vi "dfd_Build Filter Name.vi"(1 "filter name in":string) -> (0 "filter name out":string)   [LabVIEW 2017, in "NI_DigFilterLicensed.lvlib"]
uses:
  <vilib>/addons/Digital Filter Design/NI_DigFilterLicensed.lvlib
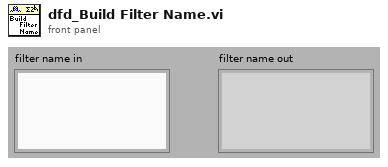
[diagram p1: front panel]
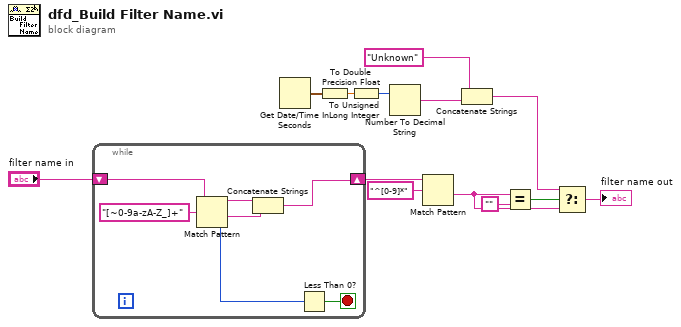
[diagram p0: block diagram]
diagram:
  n1 = while {
    shift-right: [w16] -> w3
    shift-left: "filter name in" -> [w20]
    stop <- w15 stop-if-true
    n2 = Match Pattern(string=w20, regular expression="[~0-9a-zA-Z_]+") -> (before substring=w18:string, after substring=w17:string, offset past match=w14:i32)  [unwired: 2 out]
    n3 = Concatenate Strings(w18, w17) -> (w16:string)
    n4 = Less Than 0?(x=w14) -> (x < 0?=w15:bool)
  }
  n5 = Get Date/Time In Seconds() -> (seconds since 1Jan1904=w10:timestamp)
  n6 = To Double Precision Float(number=w10) -> (double precision float=w9:dbl)
  n7 = To Unsigned Long Integer(number=w9) -> (unsigned 32bit integer=w8:u32)
  n8 = Number To Decimal String(number=w8) -> (decimal integer string=w7:string)  [unwired: 1 out]
  n9 = Match Pattern(string=w3, regular expression="^[0-9]*") -> (after substring=w1:string)  [unwired: 4 out]
  n10 = Concatenate Strings("Unknown" ("t"), w7) -> (w5:string)
  n11 = Equal?(x=w1, y="") -> (x = y?=w11:bool)
  n12 = Select(t=w5, s=w11, f=w1) -> (s? t:f=→"filter name out":string)
